vi "set_master_range_offset.vi"(8 "error in (no error)":errorcluster, 10 "range and offset":T1={"range"=7.119999645510688e-05, "offset"=0.10570889711380005} {"offset" min=0.0 max=1.0 step=0.0010000000474974513 scale=0.0..1.0; "range" min=0.0 max=1.0 step=0.0010000000474974513 scale=0.0..1.0}, 11 "DL090216RangeOffsetImageProcessor.lvclass in":refnum<class "ImageProcessorDL090216RangeOffset.lvclass">) -> (0 "error out":errorcluster, 3 "DL090216RangeOffsetImageProcessor.lvclass out":refnum<class "ImageProcessorDL090216RangeOffset.lvclass">)   [LabVIEW 2010, in "ImageProcessorDL090216RangeOffset.lvclass"]
uses:
  ImageProcessorDL090216RangeOffset.lvclass
  common/clusters/range_offset_cluster.ctl
  ImageProcessorDL090216RangeOffset.lvclass/ImageProcessorDL090216RangeOffset.ctl
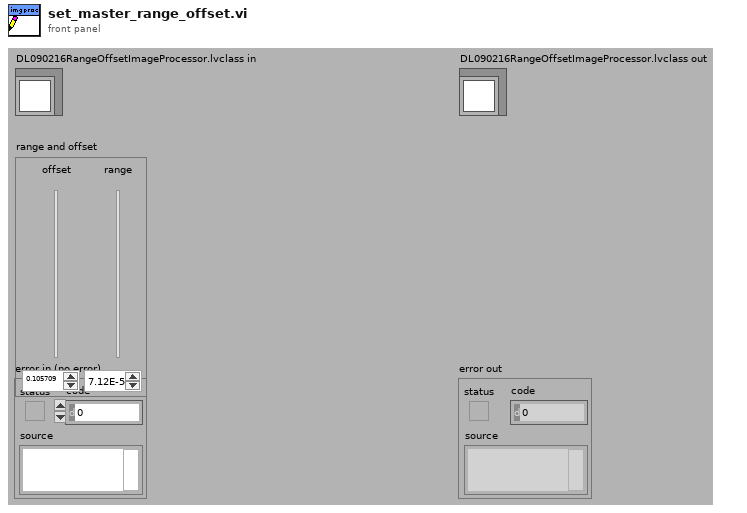
[diagram p1: front panel]
types:
  T1 = typedef "range_offset_cluster.ctl" = cluster{"range":dbl, "offset":dbl}
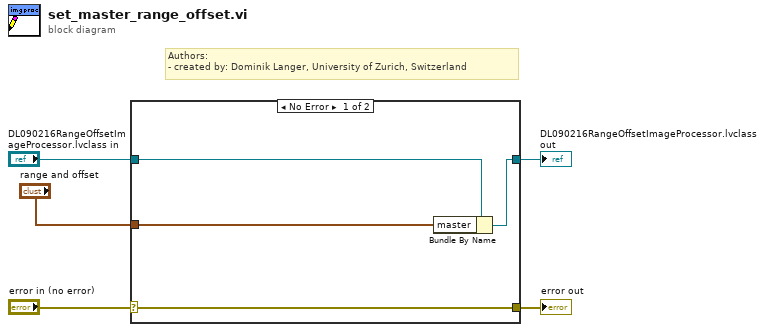
[diagram p0: block diagram]
diagram:
  # "Authors: \n- created by: Dominik Langer, University of Zurich, Switzerland"
  n1 = case shown="No Error" "error in (no error)" {
    selector: "error in (no error)" -> [w9 w10]
    tunnel: [w9 w10] -> w4
    tunnel: [w7 w11] -> w2
    tunnel: "DL090216RangeOffsetImageProcessor.lvclass in" -> [w8 w11]
    tunnel: "range and offset" -> [w6 _]
    frame No Error {
      n2 = Bundle By Name(cluster=w8, "master"=w6) -> (w7:refnum<class "ImageProcessorDL090216RangeOffset.lvclass">)
    }
    frame Error {
    }
  }
  "error out" <- w4
  "DL090216RangeOffsetImageProcessor.lvclass out" <- w2
